vi "Read Rule parser names.vi"(11 "UIManager in":refnum<class "UIManager.lvclass">) -> (1 "Rule parser names":string[](array[string]), 3 "UIManager out":refnum<class "UIManager.lvclass">)   [LabVIEW 2020, in "DependencyInspector.lvlib" / "UIManager.lvclass"]
uses:
  UIManager.lvclass
  UIManager.lvclass/UIManager.ctl
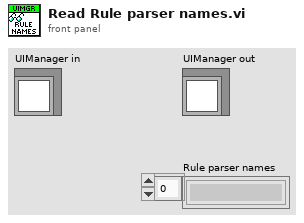
[diagram p1: front panel]
types:
  T1 = map{string, refnum<class "IRuleFileParser.lvclass">}
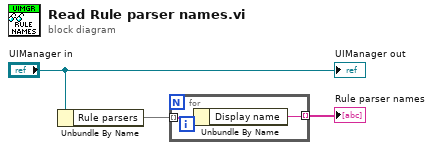
[diagram p0: block diagram]
diagram:
  n1 = Unbundle By Name("UIManager in") -> ("Rule parsers"=w2:T1)
  n2 = for {
    tunnel: w2 -> [w5] mode=indexing
    tunnel: [w4] -> w1 mode=indexing
    n3 = Unbundle By Name(w5) -> ("Display name"=w4:string)
  }
  "Rule parser names" <- w1
  "UIManager out" <- "UIManager in"
